vi "Write ZI Handle.vi"(8 "error in (no error)":errorcluster, 10 "ziHandle":T1 {"Handle" format="0x%08x"; "Conn" format="0x%08x"}, 11 "ZI Lockin in":refnum<class "ZI Lockin.lvclass">) -> (0 "error out":errorcluster, 3 "ZI Lockin out":refnum<class "ZI Lockin.lvclass">)   [LabVIEW 2016, in "ZI Lockin.lvclass"]
uses:
  ZI Lockin.lvclass
  <instrlib>/Zurich Instruments LabOne/Public/ziTypeHandle.ctl
  ZI Lockin.lvclass/ZI Lockin.ctl
  <instrlib>/Zurich Instruments LabOne/Zurich Instruments LabOne.lvlib
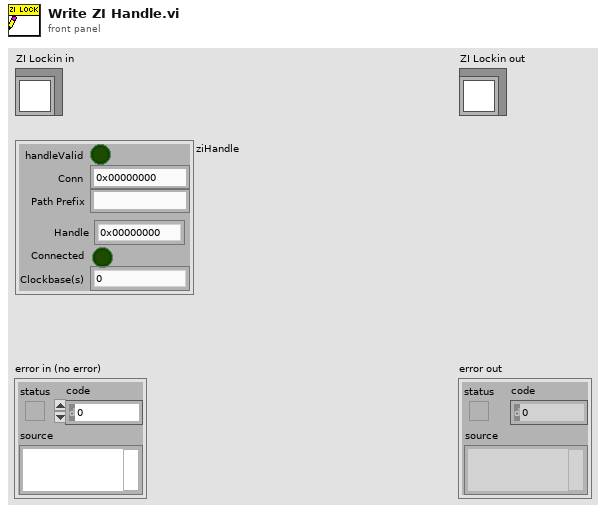
[diagram p1: front panel]
types:
  T1 = typedef "Zurich Instruments LabOne.lvlib/ziTypeHandle.ctl" = cluster{"handleValid":bool, "Conn":u64, "Path Prefix":string, "Handle":u64, "Connected":bool, "Clockbase(s)":dbl}
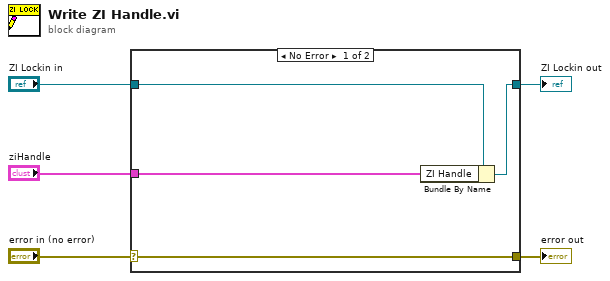
[diagram p0: block diagram]
diagram:
  n1 = case shown="No Error" "error in (no error)" {
    selector: "error in (no error)" -> [w9 w10]
    tunnel: [w9 w10] -> w4
    tunnel: [w7 w11] -> w2
    tunnel: "ZI Lockin in" -> [w8 w11]
    tunnel: "ziHandle" -> [w6 _]
    frame No Error {
      n2 = Bundle By Name(cluster=w8, "ZI Handle"=w6) -> (w7:refnum<class "ZI Lockin.lvclass">)
    }
    frame Error {
    }
  }
  "error out" <- w4
  "ZI Lockin out" <- w2
